vi "cDAQ Interpret AI Data.vi"(6 "Indexes used":i32[](array[numeric]), 8 "Setup":T2={"Test Setup"={"RH Resistor"=100.0, "Temp Resistor"=100.0, "Gas P. Resistor"=250.0, "Temp4mA Val"=32.0, "Temp20mA Val"=212.0, "RH4mA Val"=0.0, "RH20mA Val"=100.0, "GPres4mA Val"=0.0, "Gpres20mA Val"=50.0}, "cDAQ Array Locations"={"Scale Channel"=90, "TC Channels"=0, "VDC Discrete Channel"=72, "RH Chan"=91, "Temp Chan"=93, "Tscale Channel"=2, "RDB Channel"=0, "Gas Temperature"=88, "Gas Pressure"=89, "Barometric Pressure"=94, "Gas Feedback Chan"=92}}, 9 "Temp Means":dbl[](array[numeric])=[-101440.14950293404, 0.0, 0.0, 0.0, 0.0, 0.0, 0.0, 0.0, 0.0, 0.0, 0.0, 0.0, 0.0, 0.0, 0.0, 0.0, 0.0, 0.0, 0.0, 0.0, 0.0, 0.0, 0.0, 0.0, 0.0, 0.0, 0.0, 0.0, 0.0, 0.0, 0.0, 0.0, 0.0, 0.0, 0.0, 0.0, 0.0, 0.0, 0.0, 0.0, 0.0, 0.0, 0.0, 0.0, 0.0, 0.0, 0.0, 0.0, 0.0, 0.0, 0.0, 0.0, 0.0, 0.0, 0.0, 0.0, 0.0, 0.0, 0.0, 0.0, 0.0, 0.0, 0.0, 0.0, 0.0, 0.0, 0.0, 0.0, 0.0, 0.0, 0.0, 0.0, 0.0, 0.0, 0.0, 0.0, 0.0, 0.0, 0.0, 0.0, 0.0, 0.0, 0.0, 0.0, 0.0, 0.0, 0.0, 0.0, 0.0, 0.0, 0.0, 0.0, 0.0, 0.0, 0.0], 10 "Gas Temp":T1, 11 "AI Data":T1[](array[typedef])) -> (2 "cDAQ Data Out":dbl[](array[numeric]), 3 "appended array":dbl[](array[numeric]))   [LabVIEW 2014]
doc: "Converts analog input voltages to readable measurements:\nGas Pressure, RH, Temp, Barometric Pressure, Gas Volume\nAlso stores these measurements and TC meas. in output data array."
uses:
  Type Definitions/cDAQ Instrument Sensor.ctl
  Type Definitions/cDAQ Setup.ctl
panel:
  out "Labels":string[](array[string])=["Gas Pressure", "RH Channel", "Temp Channe;", "Barometric Pressure", "Gas Feedback Chan", "Gas Temperature"]
  out "Chosen temps":dbl[](array[numeric])
  in  "I.Gvol":i32=3
  in  "I.Bar":i32=5
  in  "I.Tmp":i32=4
  in  "I.RH":i32=2
  in  "I.Gas Pressure":i32
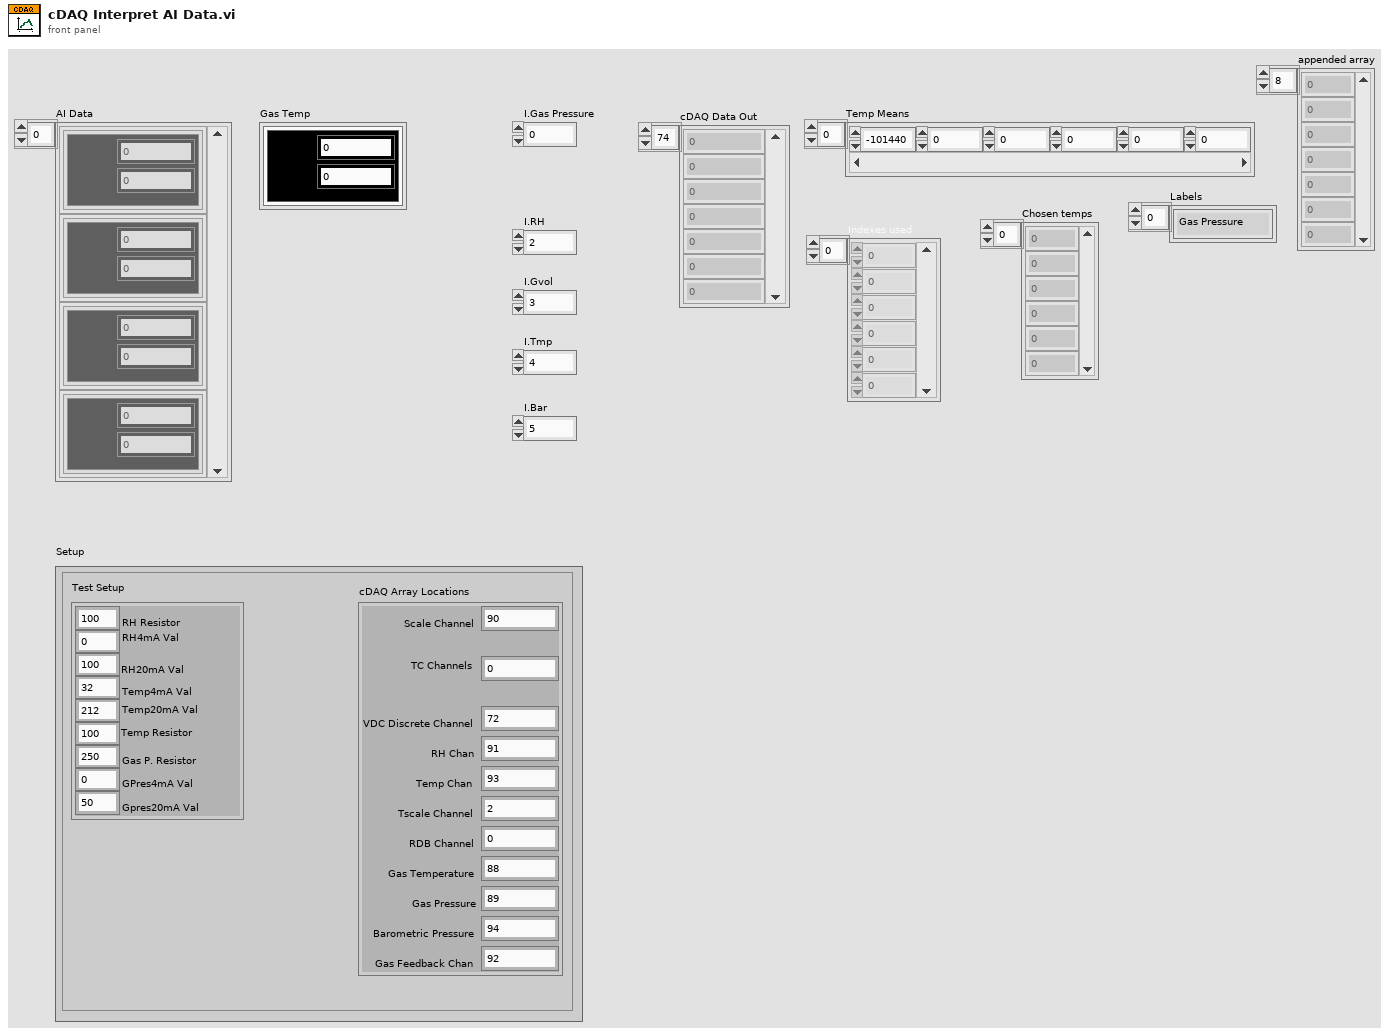
[diagram p1: front panel]
types:
  T1 = typedef "cDAQ Instrument Sensor.ctl" = cluster{"Mean":dbl, " Std":dbl, "Color Box":u32}
  T2 = typedef "cDAQ Setup.ctl" = cluster{"Test Setup":cluster{"RH Resistor":dbl, "Temp Resistor":dbl, "Gas P. Resistor":dbl, "Temp4mA Val":dbl, "Temp20mA Val":dbl, "RH4mA Val":dbl, "RH20mA Val":dbl, "GPres4mA Val":dbl, "Gpres20mA Val":dbl}, "cDAQ Array Locations":cluster{"Scale Channel":i32, "TC Channels":i32, "VDC Discrete Channel":i32, "RH Chan":i32, "Temp Chan":i32, "Tscale Channel":i32, "RDB Channel":i32, "Gas Temperature":i32, "Gas Pressure":i32, "Barometric Pressure":i32, "Gas Feedback Chan":i32}}
  T3 = cluster{"RH Resistor":dbl, "Temp Resistor":dbl, "Gas P. Resistor":dbl, "Temp4mA Val":dbl, "Temp20mA Val":dbl, "RH4mA Val":dbl, "RH20mA Val":dbl, "GPres4mA Val":dbl, "Gpres20mA Val":dbl}
  T4 = cluster{"Scale Channel":i32, "TC Channels":i32, "VDC Discrete Channel":i32, "RH Chan":i32, "Temp Chan":i32, "Tscale Channel":i32, "RDB Channel":i32, "Gas Temperature":i32, "Gas Pressure":i32, "Barometric Pressure":i32, "Gas Feedback Chan":i32}
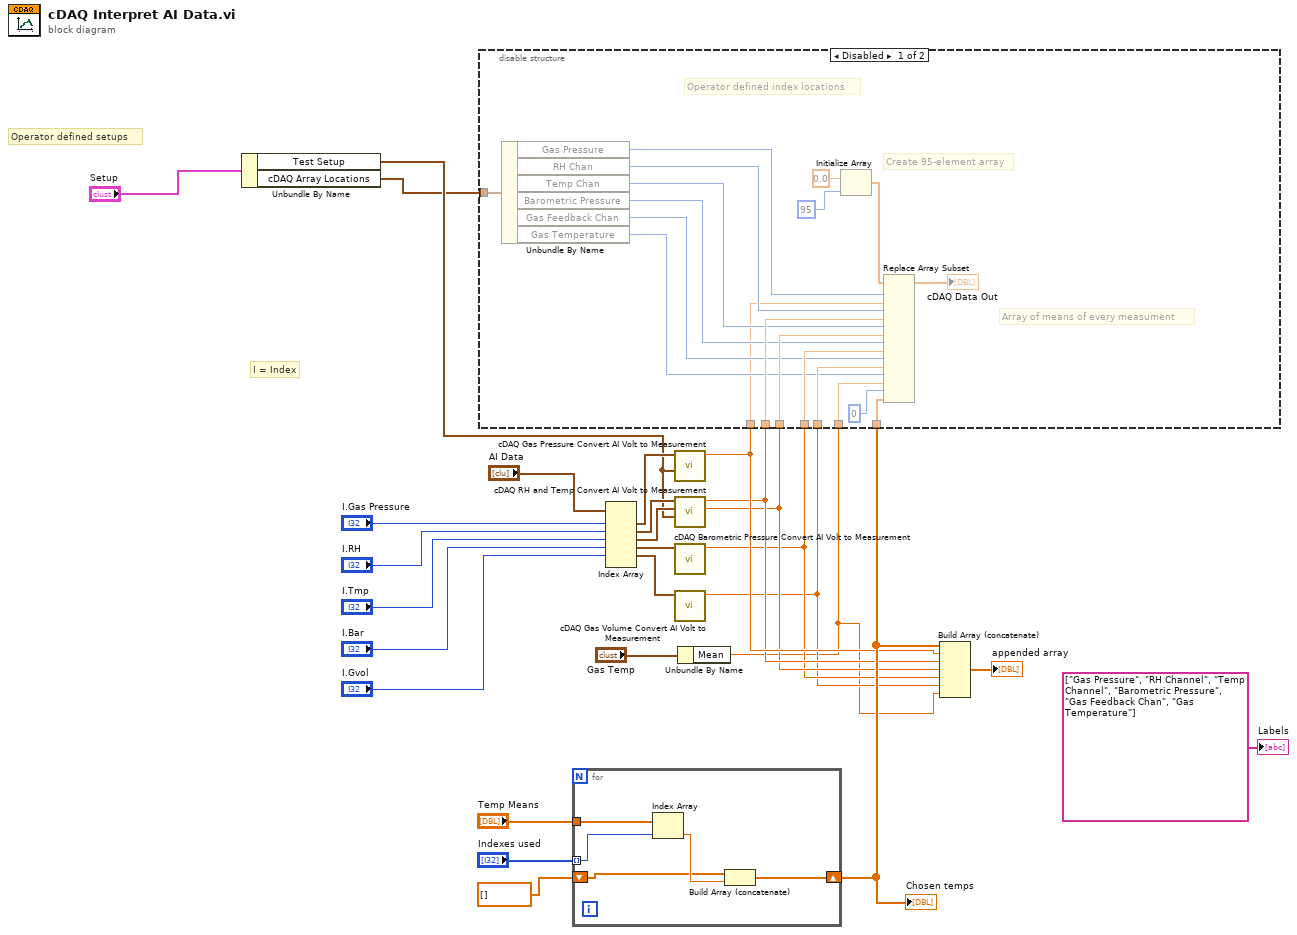
[diagram p0: block diagram]
diagram:
  # "Operator defined setups"
  # "I = Index"
  n1 = Unbundle By Name("Setup") -> ("Test Setup"=w20:T3, "cDAQ Array Locations"=w19:T4)
  n2 = for {
    tunnel: "Indexes used" -> [w31] mode=indexing
    tunnel: "Temp Means" -> [w32]
    shift-right: [w29] -> w10
    shift-left: dbl[] [] -> [w28]
    n3 = Index Array(array=w32, index=w31) -> (element=w30:dbl)
    n4 = Build Array (concatenate)(w28, w30) -> (w29:dbl[])
  }
  "Chosen temps" <- w10
  n5 = Index Array(array="AI Data", index #1="I.Gas Pressure", index #2="I.RH", index #3="I.Tmp", index #4="I.Bar", index #5="I.Gvol") -> (element #1=w23:T1, element #2=w22:T1, element #3=w21:T1, element #4=w16:T1, element #5=w15:T1)  [unwired: 1 in, 1 out]
  n6 = call "cDAQ Gas Pressure Convert AI Volt to Measurement.vi"("Test Setup"=w20, "AI Voltage"=w23) -> ("Mean measurement (in. H20)"=w9:dbl)  [unwired: 9 in]
  n7 = call "cDAQ RH and Temp Convert AI Volt to Measurement.vi"("Test Setup"=w20, "Temp Volt"=w21, "RH Volt"=w22) -> ("Temp Mean measurement (F)"=w7:dbl, "RH Mean measurement (%)"=w8:dbl)  [unwired: 7 in]
  n8 = call "cDAQ Barometric Pressure Convert AI Volt to Measurement.vi"("AI Voltage"=w16) -> ("Mean measurement (in. Hg)"=w6:dbl)  [unwired: 10 in]
  n9 = call "cDAQ Gas Volume Convert AI Volt to Measurement.vi"("AI Voltage"=w15) -> ("Mean measurement (Liters)"=w5:dbl)  [unwired: 10 in]
  n10 = Unbundle By Name("Gas Temp") -> ("Mean"=w4:dbl)
  n11 = disable-structure shown="Disabled" {
    disable-tunnel: w19 -> [w51 _]
    disable-tunnel: w8 -> [w50 _]
    disable-tunnel: w7 -> [w49 _]
    disable-tunnel: w6 -> [w48 _]
    disable-tunnel: w5 -> [w47 _]
    disable-tunnel: w9 -> [w39 _]
    disable-tunnel: w4 -> [w35 _]
    disable-tunnel: w10 -> [w33 _]
    frame Disabled {
      # "Create 95-element array"
      # "Operator defined index locations"
      # "Array of means of every measument"
      n12 = Unbundle By Name(w51) -> ("Gas Pressure"=w41:i32, "RH Chan"=w42:i32, "Temp Chan"=w40:i32, "Barometric Pressure"=w43:i32, "Gas Feedback Chan"=w44:i32, "Gas Temperature"=w45:i32)
      n13 = Initialize Array(0.0 ("element"), 95 ("dimension size")) -> (w36:dbl[])
      n14 = Replace Array Subset(array=w36, new element #1=w39, index #1=w41, new element #2=w50, index #2=w42, new element #3=w49, index #3=w40, new element #4=w48, index #4=w43, new element #5=w47, index #5=w44, new element #6=w35, index #6=w45, new element #7=w33, index #7=0 ("index")) -> (→"cDAQ Data Out":dbl[])
    }
    frame Enabled {
    }
  }
  n15 = Build Array (concatenate)(w10, w9, w8, w7, w6, w5, w4) -> (→"appended array":dbl[])
  "Labels" <- string[] ["Gas Pressure", "RH Channel", "Temp Channel", "Barometric Pressure", "Gas Feedback Chan", "Gas Temperature"]
